vi "myAppView.vi"() -> ()   [LabVIEW 2013, in "myAppView.lvclass"]
uses:
  myAppView.lvclass
  Framework/View/base/VIEW.lvclass
  Framework/Controller/base/CONTROLLER.lvclass
panel:
  in  "error in":errorcluster
  out "error out":errorcluster
  in  "Numeric Control":dbl
  in  "stop":bool
  in  "ctrl2":string
  in  "DoAction1":bool
  in  "Enqueue Element":bool
  in  "mystring":string
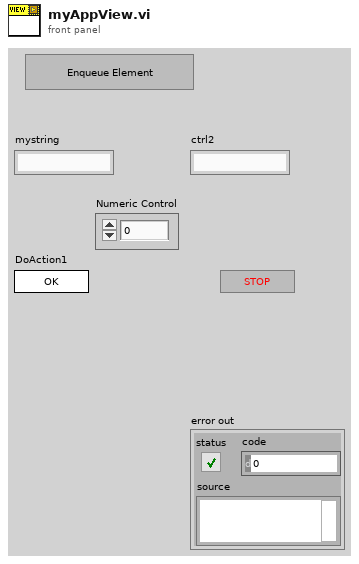
[diagram p1: front panel]
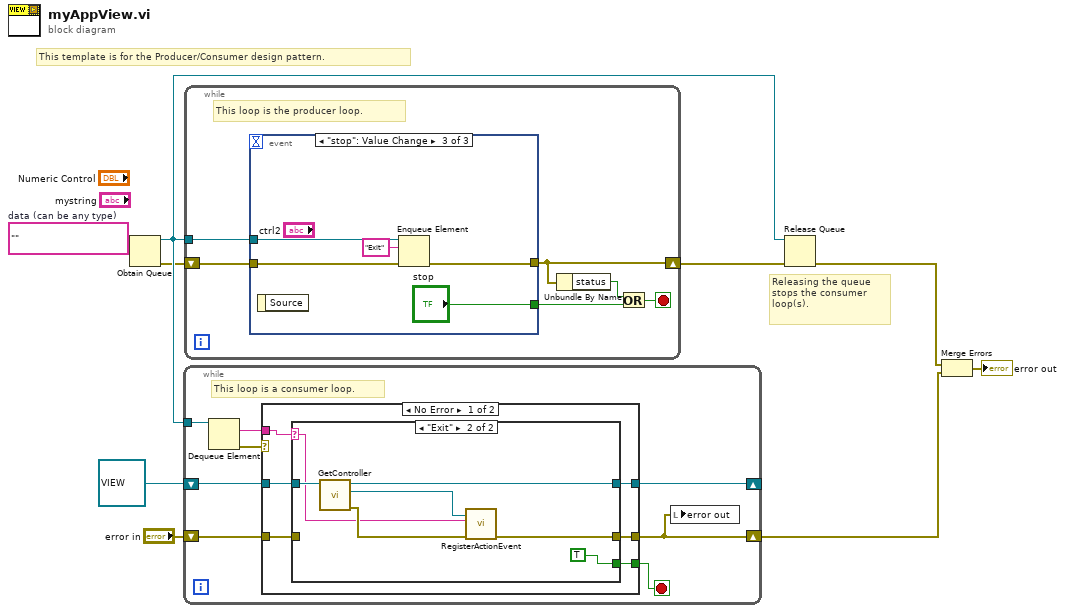
[diagram p0: block diagram]
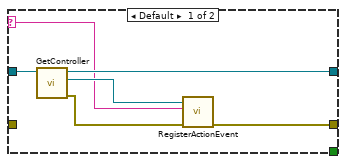
[diagram p2: hidden frame]
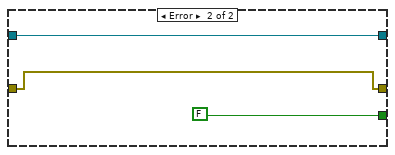
[diagram p3: hidden frame]
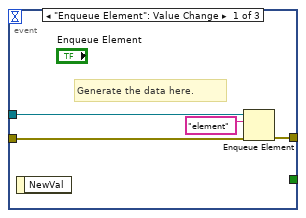
[diagram p4: hidden frame]
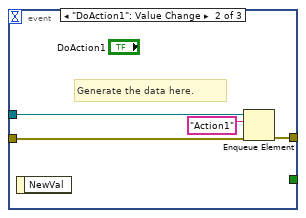
[diagram p5: hidden frame]
diagram:
  w7 = ""  # data (can be any type)
  # "Releasing the queue stops the consumer loop(s)."
  # "This template is for the Producer/Consumer design pattern."
  n1 = Obtain Queue(element data type=w7) -> (queue out=w8:refnum<queue>, error out=w5:errorcluster)  [unwired: 4 in, 1 out]
  n2 = while {
    tunnel: w8 -> [w17]
    shift-right: [w12] -> _
    shift-left: refnum<class "VIEW.lvclass"> refnum ("VIEW.lvclass") -> [w13]
    shift-right: [w10] -> w3
    shift-left: "error in" -> [w11]
    stop <- w14 stop-if-true
    # "This loop is a consumer loop."
    n3 = Dequeue Element(queue=w17) -> (element=w15:string, error out=w16:errorcluster)  [unwired: 2 in, 2 out]
    n4 = case shown="No Error" w16 {
      tunnel: w15 -> [w23 _]
      tunnel: [w20 FALSE] -> w14
      tunnel: w13 -> [w22 w38]
      tunnel: [w21 w38] -> w12
      tunnel: [w19 w37] -> w10
      tunnel: w11 -> [w18 w37]
      frame No Error {
        n5 = case shown="\"Exit\"" w23 {
          selector: w23 -> [w24 w30]
          tunnel: w22 -> [w29 w36]
          tunnel: [w27 w34] -> w21
          tunnel: [_ TRUE] -> w20
          tunnel: [w26 w31] -> w19
          tunnel: w18 -> [_ _]
          frame Default {
            n6 = call-dynamic "GetController.vi"("VIEW in"=w29) -> ("error out"=w25:errorcluster, "CONTROLLER"=w28:refnum<class "CONTROLLER.lvclass">, "VIEW out"=w27:refnum<class "VIEW.lvclass">)  [unwired: 8 in]
            n7 = call "RegisterActionEvent.vi"("error in (no error)"=w25, "Action"=w24, "CONTROLLER in"=w28) -> ("error out"=w26:errorcluster)  [unwired: 7 in, 1 out]
          }
          frame "Exit" {
            n8 = call-dynamic "GetController.vi"("VIEW in"=w36) -> ("error out"=w32:errorcluster, "CONTROLLER"=w35:refnum<class "CONTROLLER.lvclass">, "VIEW out"=w34:refnum<class "VIEW.lvclass">)  [unwired: 8 in]
            n9 = call "RegisterActionEvent.vi"("error in (no error)"=w32, "Action"=w30, "CONTROLLER in"=w35) -> ("error out"=w31:errorcluster)  [unwired: 7 in, 1 out]
          }
        }
      }
      frame Error {
      }
    }
    n10 = local write "error out"(w10) -> ()
  }
  n11 = while {
    shift-right: [w41] -> w6
    shift-left: w5 -> [w44]
    tunnel: w8 -> [w45]
    stop <- w42 stop-if-true
    # "This loop is the producer loop."
    n12 = event shown="[2] \"stop\": Value Change" {
      selector: _ -> [_ _ _]
      dyn-events: _ -> [_ _ _]
      timeout: _ -> [_ _ _]
      tunnel: w45 -> [w49 w53 w55]
      tunnel: w44 -> [w48 w52 w57]
      tunnel: [w47 w51 w56] -> w41
      tunnel: [_ _ "stop"] -> w43
      event "Enqueue Element": Value Change {
        # "Generate the data here."
        n13 = event-data() -> ()  [unwired: 1 in, 1 out]
        n14 = Enqueue Element(queue=w49, element="element", error in (no error)=w48) -> (error out=w47:errorcluster)  [unwired: 1 in, 2 out]
      }
      event "DoAction1": Value Change {
        # "Generate the data here."
        n15 = event-data() -> ()  [unwired: 1 in, 1 out]
        n16 = Enqueue Element(queue=w53, element="Action1", error in (no error)=w52) -> (error out=w51:errorcluster)  [unwired: 1 in, 2 out]
      }
      event "stop": Value Change {
        n17 = event-data() -> ()  [unwired: 1 in, 1 out]
        n18 = Enqueue Element(queue=w55, element="Exit", error in (no error)=w57) -> (error out=w56:errorcluster)  [unwired: 1 in, 2 out]
      }
    }
    n19 = Unbundle By Name(w41) -> ("status"=w40:bool)
    n20 = Or(x=w40, y=w43) -> (x .or. y?=w42:bool)
  }
  n21 = Release Queue(queue=w8, error in (no error)=w6) -> (error out=w4:errorcluster)  [unwired: 1 in, 2 out]
  n22 = Merge Errors(w4, w3) -> (→"error out":errorcluster)
